vi "task4_sine_cosine.vi"() -> ()   [LabVIEW 2020]
panel:
  out "Waveform Chart":cluster{dbl, dbl}(graph)
  out "y2":dbl
  out "y1":dbl
  in  "stop":bool
  in  "phi2":dbl
  in  "omega2":dbl
  in  "A2":dbl
  in  "phi1":dbl
  in  "omega1":dbl
  in  "A1":dbl
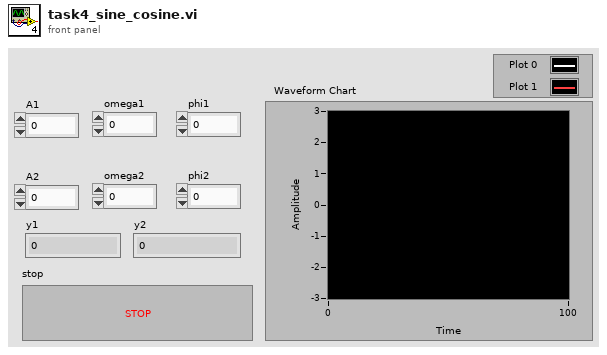
[diagram p1: front panel]
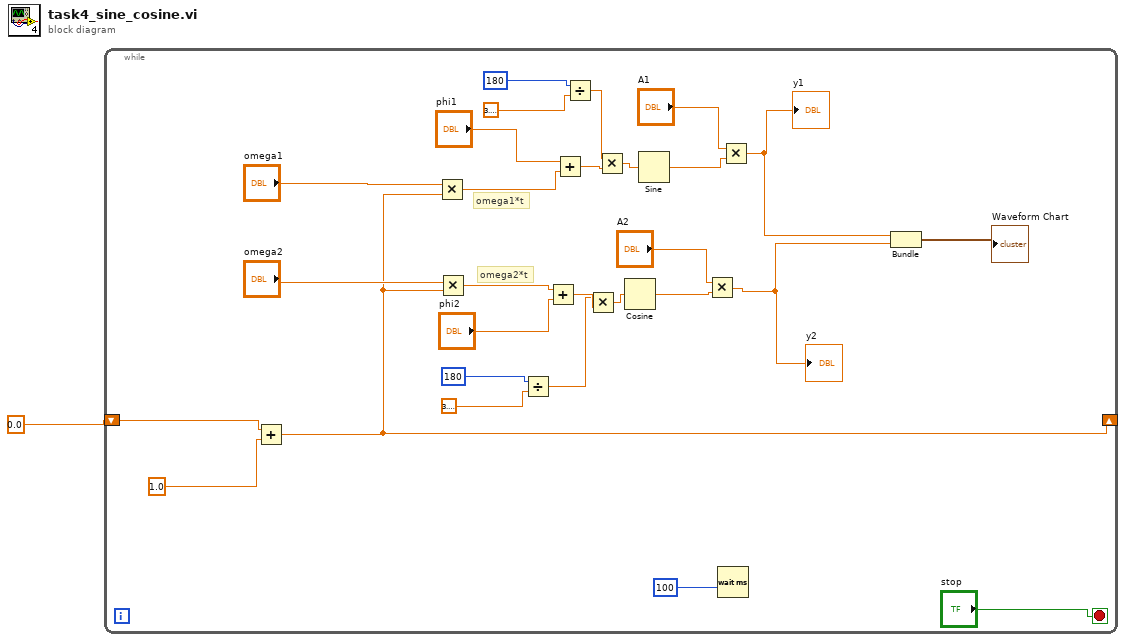
[diagram p0: block diagram]
diagram:
  n1 = while {
    shift-right: [w19] -> _
    shift-left: 0.0 -> [w28]
    stop <- "stop" stop-if-true
    # "omega1*t"
    # "omega2*t"
    n2 = Add(x=w28, y=1.0) -> (x+y=w19:dbl)
    n3 = Multiply(x="omega1", y=w19) -> (x*y=w21:dbl)
    n4 = Multiply(x="omega2", y=w19) -> (x*y=w23:dbl)
    n5 = Divide(x=180, y=3.141592653589793) -> (x/y=w2:dbl)
    n6 = Add(x=w23, y="phi2") -> (x+y=w3:dbl)
    n7 = Add(x="phi1", y=w21) -> (x+y=w6:dbl)
    n8 = Divide(x=180, y=3.141592653589793) -> (x/y=w5:dbl)
    n9 = Multiply(x=w2, y=w3) -> (x*y=w4:dbl)
    n10 = Multiply(x=w5, y=w6) -> (x*y=w7:dbl)
    n11 = Cosine(x=w4) -> (cos(x)=w17:dbl)
    n12 = Sine(x=w7) -> (sin(x)=w16:dbl)
    n13 = Multiply(x="A2", y=w17) -> (x*y=w13:dbl)
    "y2" <- w13
    n14 = Wait (ms)(milliseconds to wait=100) -> ()  [unwired: 1 out]
    n15 = Multiply(x="A1", y=w16) -> (x*y=w14:dbl)
    "y1" <- w14
    n16 = Bundle(w14, w13) -> (→"Waveform Chart":cluster{dbl, dbl})  [unwired: 1 in]
  }
